vi "xijk_give_warning_brightness.vi"(8 "error in":errorcluster, 9 "brightness 2 in":dbl, 10 "Number of fluorophores":u16(ring)=1 items=["1", "2"], 11 "brightness 1 in":dbl) -> (0 "error out":errorcluster)   [LabVIEW 2010]
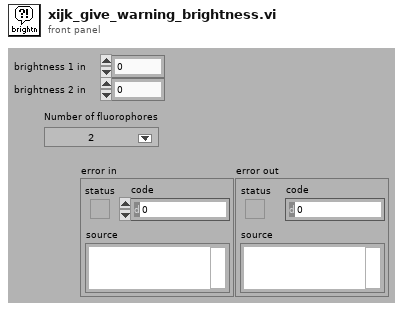
[diagram p1: front panel]
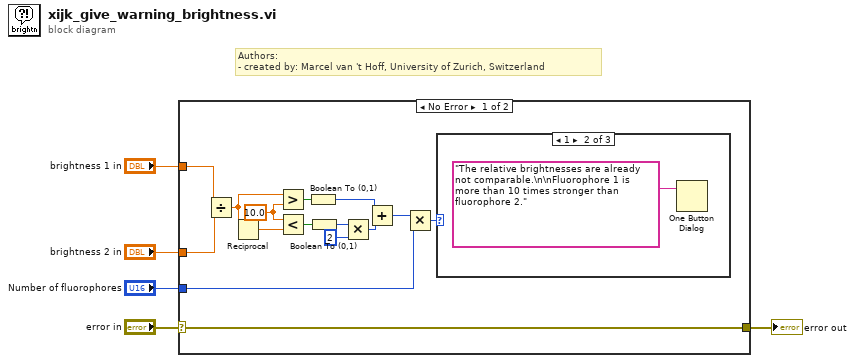
[diagram p0: block diagram]
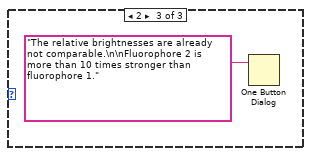
[diagram p3: hidden frame]
diagram:
  # "Authors: \n- created by: Marcel van 't Hoff, University of Zurich, Switzerland"
  n1 = case shown="No Error" "error in" {
    selector: "error in" -> [w9 w23]
    tunnel: "brightness 2 in" -> [w20 _]
    tunnel: "brightness 1 in" -> [w19 _]
    tunnel: [w9 w23] -> w2
    tunnel: "Number of fluorophores" -> [w8 _]
    frame No Error {
      w12 = 10.0 ("y")
      n2 = Divide(x=w19, y=w20) -> (x/y=w10:dbl)
      n3 = Reciprocal(x=w10) -> (1/x=w11:dbl)
      n4 = Greater?(x=w10, y=w12) -> (0:w13:bool)
      n5 = Less?(x=w12, y=w11) -> (x < y?=w14:bool)
      n6 = Boolean To (0,1)(Boolean=w13) -> (0, 1=w18:i16)
      n7 = Boolean To (0,1)(Boolean=w14) -> (0, 1=w15:i16)
      n8 = Multiply(x=w15, y=i16 2) -> (x*y=w17:i16)
      n9 = Add(x=w18, y=w17) -> (x+y=w6:i16)
      n10 = Multiply(x=w6, y=w8) -> (x*y=w7:u16)
      n11 = case shown="1" w7 {
        frame 0, Default {
        }
        frame 1 {
          n12 = One Button Dialog(message="The relative brightnesses are already not comparable.\n\nFluorophore 1 is more than 10 times stronger than fluorophore 2.") -> ()  [unwired: 2 out]
        }
        frame 2 {
          n13 = One Button Dialog(message="The relative brightnesses are already not comparable.\n\nFluorophore 2 is more than 10 times stronger than fluorophore 1.") -> ()  [unwired: 2 out]
        }
      }
    }
    frame Error {
    }
  }
  "error out" <- w2
